vi "Find and Rank Suggestions.vi"(9 "Suggestion Limit (-1: No limit)":i32=-1, 10 "Query":string, 11 "Keywords":string[](array[string])) -> (1 "Match?":bool, 3 "Suggestions":T1[](array[typedef]))   [LabVIEW 2016, in "Suggestion Box.lvclass"]
doc: "Searches for <b>Suggestions</b> in <b>Keywords</b> for the given <b>Query</b> and ranks them in order of increasing Levenshtein Distance.\n<b>Match Offsets</b> returns the character indices in <b>Keywords</b> where <b>Query</b> was found to match.\n<b>Match?</b> will be True if <b>Suggestions</b> is not an empty array.\n--------------------\nCopyright (c) 2019 Analog Devices, Inc. All rights reserved.\n\nRedistribution and use in source and binary forms, with or without modification,\nare permitted provided that the following conditions are met:\n - Redistributions of source code must retain the above copyright notice, this\n list of conditions and the following disclaimer.\n - Redistributions in binary form must reproduce the above copyright notice,\n this list of conditions and the following disclaimer in the documentation\n and/or other materials provided with the distribution.\n - Modified versions of the software must be conspicuously marked as such.\n - This software is licensed solely and exclusively for use with\n processors/products manufactured by or for Analog Devices, Inc.\n - This software may not be combined or merged with other code in any manner\n that would cause the software to become subject to terms and conditions\n which differ from those listed here.\n - Neither the name of Analog Devices, Inc. nor the names of its contributors\n may be used to endorse or promote products derived from this software\n without specific prior written permission.\n - The use of this software may or may not infringe the patent rights of one or\n more patent holders. This license does not release you from the requirement\n that you obtain separate licenses from these patent holders to use this\n software.\n\nTHIS SOFTWARE IS PROVIDED BY ANALOG DEVICES, INC. AND CONTRIBUTORS \"AS IS\" AND\nANY EXPRESS OR IMPLIED WARRANTIES, INCLUDING, BUT NOT LIMITED TO,\nNON-INFRINGEMENT, TITLE, MERCHANTABILITY AND FITNESS FOR A PARTICULAR PURPOSE\nARE DISCLAIMED. IN NO EVENT SHALL ANALOG DEVICES, INC. OR CONTRIBUTORS BE LIABLE\nFOR ANY DIRECT, INDIRECT, INCIDENTAL, SPECIAL, EXEMPLARY, PUNITIVE OR\nCONSEQUENTIAL DAMAGES (INCLUDING, BUT NOT LIMITED TO, DAMAGES ARISING OUT OF\nCLAIMS OF INTELLECTUAL PROPERTY RIGHTS INFRINGEMENT; PROCUREMENT OF SUBSTITUTE\nGOODS OR SERVICES; LOSS OF USE, DATA, OR PROFITS; OR BUSINESS INTERRUPTION)\nHOWEVER CAUSED AND ON ANY THEORY OF LIABILITY, WHETHER IN CONTRACT, STRICT\nLIABILITY, OR TORT (INCLUDING NEGLIGENCE OR OTHERWISE) ARISING IN ANY WAY OUT OF\nTHE USE OF THIS SOFTWARE, EVEN IF ADVISED OF THE POSSIBILITY OF SUCH DAMAGE.\n\n2019-01-10-7CBSD SLA"
uses:
  Suggestion Box.lvclass
  String Match.ctl
  Segment.ctl
panel:
  # "Copyright (c) 2019 Analog Devices, Inc.  All rights reserved.\n\nRedistribution and use in source and binary forms, with or without modification,\nare permitted provided that the following conditions are met:\n  - Redistributions of source code must retain the above copyright notice, this\n    list of conditions and the following disclaimer.\n  - Redistributions in binary form must reproduce the above copyright notice,\n    this list of conditions and the following disclaimer in the documentation\n    and/or other materials provided with the distribution.\n  - Modified versions of the software must be conspicuously marked as such.\n  - This software is licensed solely and exclusively for use with\n    processors/products manufactured by or for Analog Devices, Inc.\n  - This software may not be combined or merged with other code in any manner\n    that would cause the software to become subject to terms and conditions\n    which differ from those listed here.\n  - Neither the name of Analog Devices, Inc. nor the names of its contributors\n    may be used to endorse or promote products derived from this software\n    without specific prior written permission.\n  - The use of this software may or may not infringe the patent rights of one or\n    more patent holders.  This license does not release you from the requirement\n    that you obtain separate licenses from these patent holders to use this\n    software.\n\nTHIS SOFTWARE IS PROVIDED BY ANALOG DEVICES, INC. AND CONTRIBUTORS \"AS IS\" AND\nANY EXPRESS OR IMPLIED WARRANTIES, INCLUDING, BUT NOT LIMITED TO,\nNON-INFRINGEMENT, TITLE, MERCHANTABILITY AND FITNESS FOR A PARTICULAR PURPOSE\nARE DISCLAIMED. IN NO EVENT SHALL ANALOG DEVICES, INC. OR CONTRIBUTORS BE LIABLE\nFOR ANY DIRECT, INDIRECT, INCIDENTAL, SPECIAL, EXEMPLARY, PUNITIVE OR\nCONSEQUENTIAL DAMAGES (INCLUDING, BUT NOT LIMITED TO, DAMAGES ARISING OUT OF\nCLAIMS OF INTELLECTUAL PROPERTY RIGHTS INFRINGEMENT; PROCUREMENT OF SUBSTITUTE\nGOODS OR SERVICES; LOSS OF USE, DATA, OR PROFITS; OR BUSINESS INTERRUPTION)\nHOWEVER CAUSED AND ON ANY THEORY OF LIABILITY, WHETHER IN CONTRACT, STRICT\nLIABILITY, OR TORT (INCLUDING NEGLIGENCE OR OTHERWISE) ARISING IN ANY WAY OUT OF\nTHE USE OF THIS SOFTWARE, EVEN IF ADVISED OF THE POSSIBILITY OF SUCH DAMAGE.\n\n2019-01-10-7CBSD SLA"
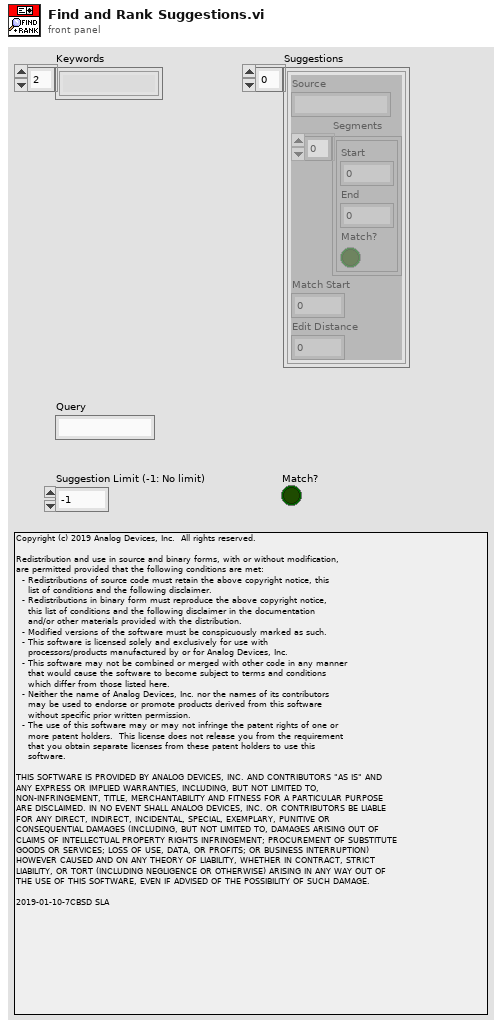
[diagram p1: front panel]
types:
  T1 = typedef "Suggestion Box.lvclass/String Match.ctl" = cluster{"Source":string, "Segments":T2[], "Match Start":i32, "Edit Distance":i32}
  T2 = typedef "Suggestion Box.lvclass/Segment.ctl" = cluster{"Start":i32, "End":i32, "Match?":bool}
  T3 = cluster{"Distance":i32, "Match Start":i32, "Index":i32}
  T4 = cluster{"Distance":i32, "Match Start":i32, "Index":i32}[]
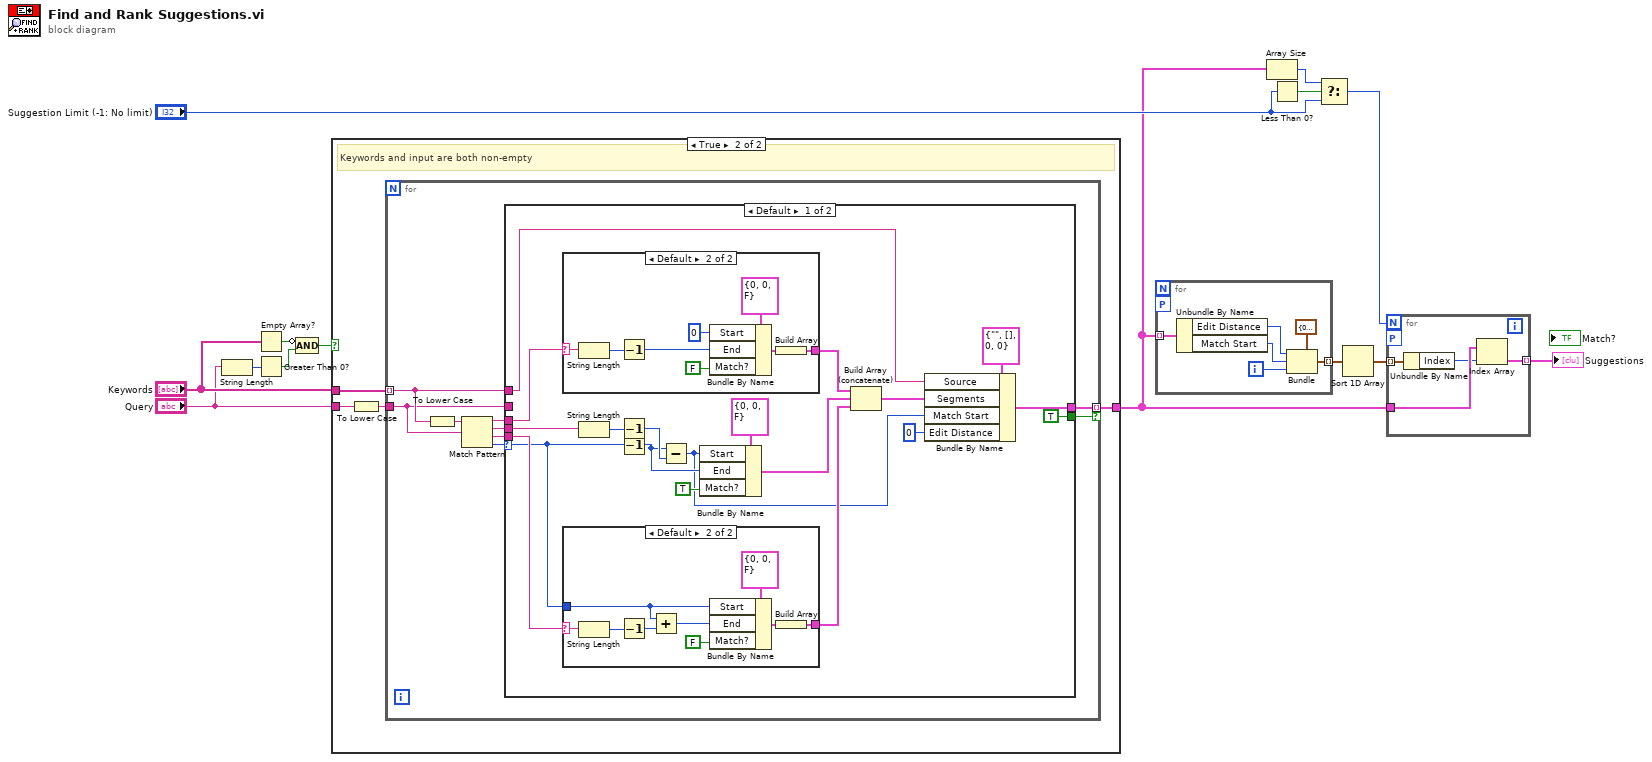
[diagram p0: block diagram]
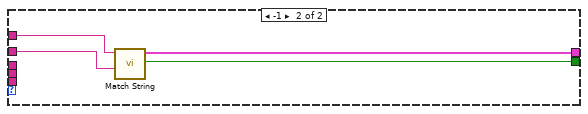
[diagram p5: hidden frame]
diagram:
  n1 = String Length(string="Query") -> (length=w12:i32)
  n2 = Empty Array?(array="Keywords") -> (empty?=w8:bool)
  n3 = Greater Than 0?(x=w12) -> (x > 0?=w14:bool)
  n4 = Compound Arithmetic op=AND(invert w8, w14) -> (w13:bool)
  n5 = case shown="True" w13 {
    tunnel: "Query" -> [_ w17]
    tunnel: "Keywords" -> [_ w18]
    tunnel: [_ w16] -> w3
    frame False {
      # "Empty Keywords or Input -- no processing needed and no suggestions to return"
    }
    frame True {
      # "Keywords and input are both non-empty"
      n6 = To Lower Case(string=w17) -> (all lower case string=w15:string)
      n7 = for {
        tunnel: w18 -> [w22] mode=indexing
        tunnel: w15 -> [w20]
        tunnel: [w27] -> w16 mode=indexing if=w19
        n8 = To Lower Case(string=w22) -> (all lower case string=w21:string)
        n9 = Match Pattern(string=w21, regular expression=w20) -> (before substring=w23:string, match substring=w24:string, after substring=w25:string, offset past match=w26:i32)  [unwired: 1 in]
        n10 = case shown="Default" w26 {
          selector: w26 -> [w36 _]
          tunnel: [w33 w67] -> w27
          tunnel: [TRUE ("Match?") w64] -> w19
          tunnel: w20 -> [_ w66]
          tunnel: w22 -> [w29 w65]
          tunnel: w25 -> [w38 _]
          tunnel: w24 -> [w37 _]
          tunnel: w23 -> [w34 _]
          frame Default {
            n11 = case shown="Default" w34 {
              selector: w34 -> [_ w51]
              tunnel: [_ w49] -> w35
              frame "" {
              }
              frame Default {
                n12 = String Length(string=w51) -> (length=w52:i32)
                n13 = Decrement(x=w52) -> (x-1=w48:i32)
                n14 = Bundle By Name(cluster=T2 {"Start"=0, "End"=0, "Match?"=FALSE} ("Segments"), "Start"=0, "End"=w48, "Match?"=FALSE) -> (w50:T2)
                n15 = Build Array(w50) -> (w49:T2[])
              }
            }
            n16 = case shown="Default" w38 {
              selector: w38 -> [_ w60]
              tunnel: w36 -> [_ w58]
              tunnel: [_ w56] -> w41
              frame "" {
              }
              frame Default {
                n17 = String Length(string=w60) -> (length=w61:i32)
                n18 = Decrement(x=w61) -> (x-1=w59:i32)
                n19 = Add(x=w58, y=w59) -> (x+y=w55:i32)
                n20 = Bundle By Name(cluster=T2 {"Start"=0, "End"=0, "Match?"=FALSE} ("Segments"), "Start"=w58, "End"=w55, "Match?"=FALSE) -> (w57:T2)
                n21 = Build Array(w57) -> (w56:T2[])
              }
            }
            n22 = String Length(string=w37) -> (length=w31:i32)
            n23 = Decrement(x=w31) -> (x-1=w46:i32)
            n24 = Decrement(x=w36) -> (x-1=w45:i32)
            n25 = Subtract(x=w45, y=w46) -> (x-y=w32:i32)
            n26 = Bundle By Name(cluster=T2 {"Start"=0, "End"=0, "Match?"=FALSE} ("Segments"), "Start"=w32, "End"=w45, "Match?"=TRUE) -> (w42:T2)
            n27 = Build Array (concatenate)(w35, w42, w41) -> (w44:T2[])
            n28 = Bundle By Name(cluster=T1 {"Source"="", "Segments"=[], "Match Start"=0, "Edit Distance"=0} ("String Match"), "Source"=w29, "Segments"=w44, "Match Start"=w32, "Edit Distance"=0) -> (w33:T1)
          }
          frame -1 {
            n29 = call "Match String.vi"("Pattern"=w66, "Source"=w65) -> ("Match?"=w64:bool, "String Match"=w67:T1)  [unwired: 8 in]
          }
        }
      }
    }
  }
  n30 = for {
    tunnel: [w73] -> w1 mode=indexing
    workers-P: _ -> [_]
    tunnel: w3 -> [w71] mode=indexing
    i -> [w72]
    n31 = Unbundle By Name(w71) -> ("Edit Distance"=w68:i32, "Match Start"=w70:i32)
    n32 = Bundle(cluster=T3 {"Distance"=0, "Match Start"=0, "Index"=0}, "Distance"=w68, "Match Start"=w70, "Index"=w72) -> (w73:T3)
  }
  n33 = Array Size(array=w3) -> (size(s)=w10:i32)
  n34 = Less Than 0?(x="Suggestion Limit (-1: No limit)") -> (x < 0?=w11:bool)
  n35 = Select(t=w10, s=w11, f="Suggestion Limit (-1: No limit)") -> (s? t:f=w4:i32)
  n36 = Sort 1D Array(array=w1) -> (sorted array=w5:T4)
  n37 = for {
    N: w4 -> [_]
    workers-P: _ -> [_]
    tunnel: w5 -> [w75] mode=indexing
    tunnel: w3 -> [w77]
    tunnel: [w76] -> w2 mode=indexing
    n38 = Unbundle By Name(w75) -> ("Index"=w74:i32)
    n39 = Index Array(array=w77, index=w74) -> (element=w76:T1)
  }
  "Suggestions" <- w2
